vi "CH0_write_byte_data_and_sign_into_mem_no_g_Rev01.vi"(0 "MB data":u8, 1 "UB data":u8, 2 "Sign addrss 8 byte":string, 3 "USB Interface Name":refnum<visa-resource-name>="COM3", 4 "HB data":u8, 5 "LB data":u8, 6 "MB addrss 8 byte":string, 7 "HB addrss 8 byte":string, 8 "Sign data 3 byte":dbl, 9 "WRITE DATA":bool, 10 "Input buffer size":u32=16384, 11 "LB addrss 8 byte":string, 12 "UB addrss 8 byte":string, 13 "error in (no error)":errorcluster, 16 "Enable memory wright":bool) -> (14 "MB data 3 byte":string, 15 "UB data 3 byte":string, 17 "error out":errorcluster, 18 "HB data 3 byte":string, 19 "LB data 3 byte":string)   [LabVIEW 2012]
panel:
  out "Reply":string
  out "T command Bytes sent 5":dbl
  out "T command Bytes sent 4":dbl
  out "T command Bytes sent 3":dbl
  out "T command Bytes sent 2":dbl
  out "T command Bytes sent":dbl
  out "First 'T' Number of bytes written":dbl
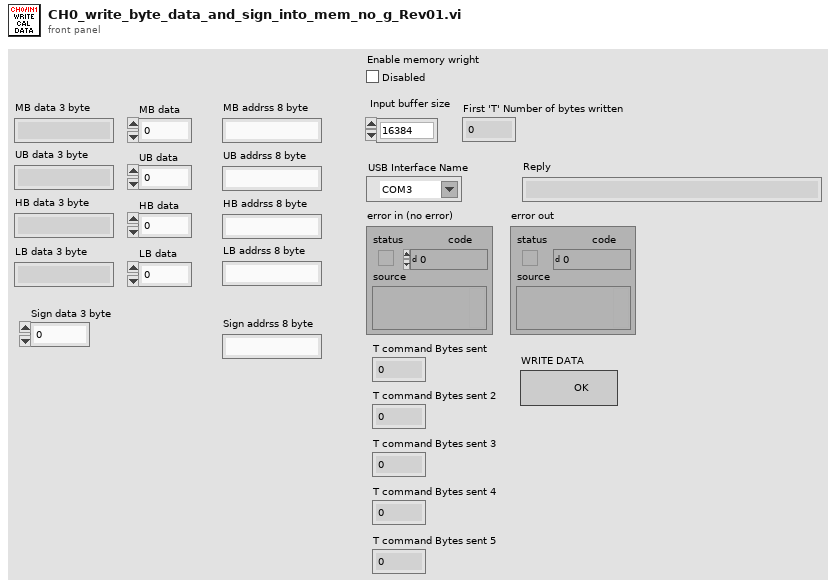
[diagram p1: front panel]
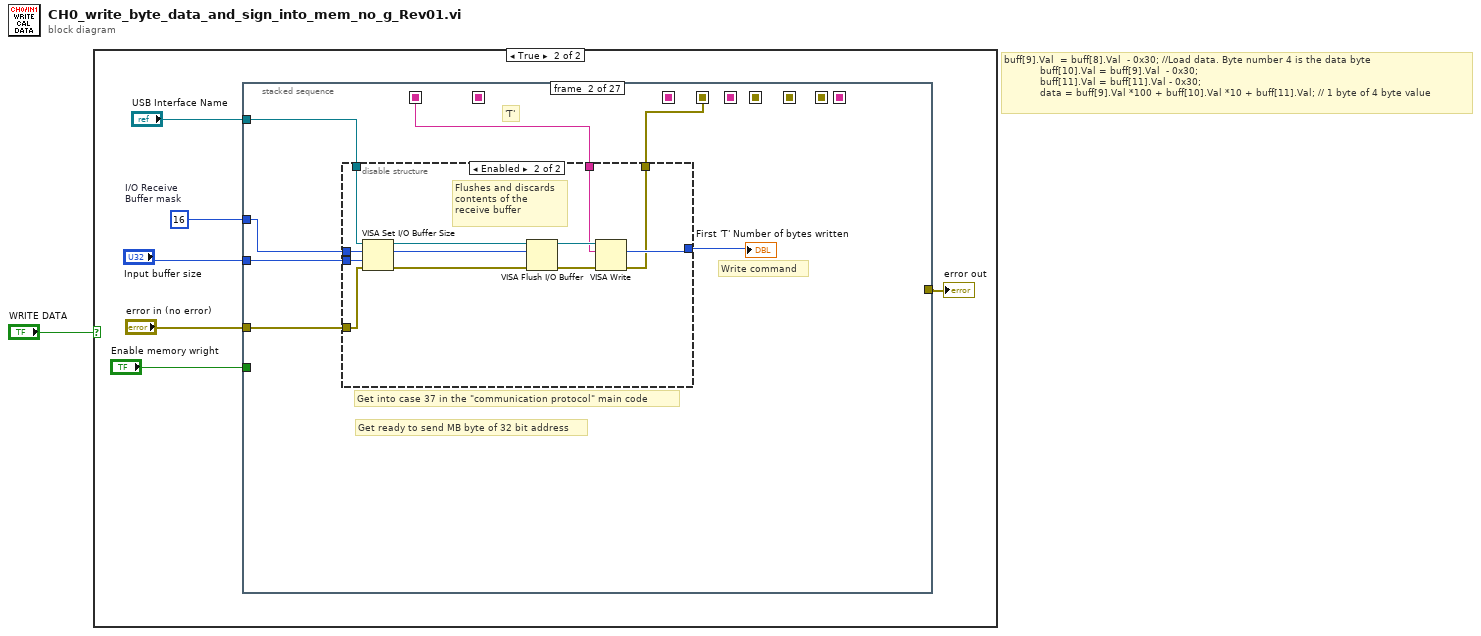
[diagram p0: block diagram]
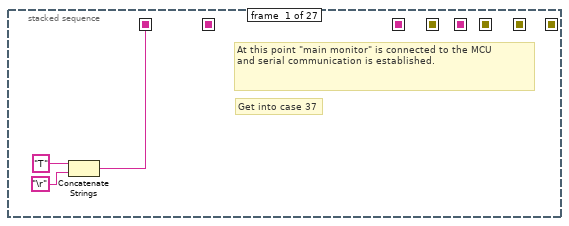
[diagram p3: hidden frame]
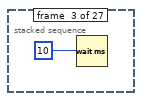
[diagram p5: hidden frame]
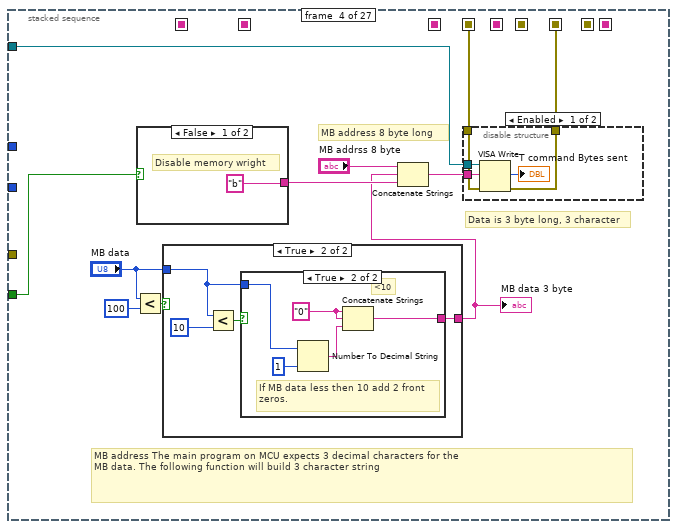
[diagram p6: hidden frame]
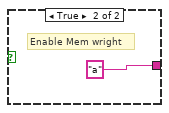
[diagram p7: hidden frame]
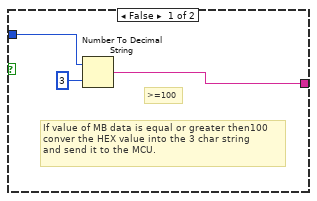
[diagram p8: hidden frame]
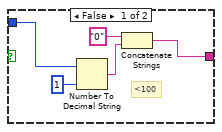
[diagram p9: hidden frame]
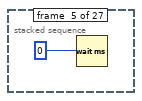
[diagram p11: hidden frame]
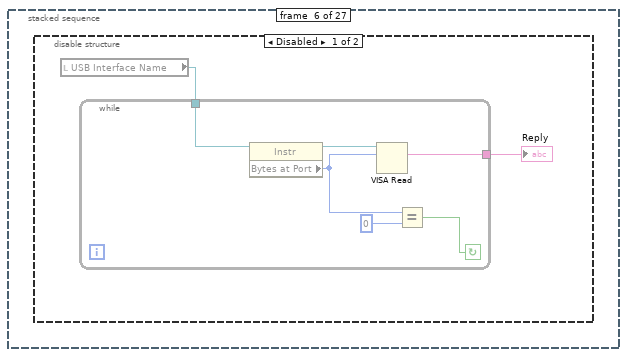
[diagram p12: hidden frame]
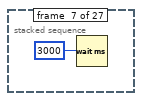
[diagram p14: hidden frame]
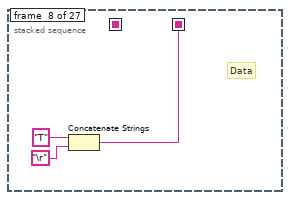
[diagram p15: hidden frame]
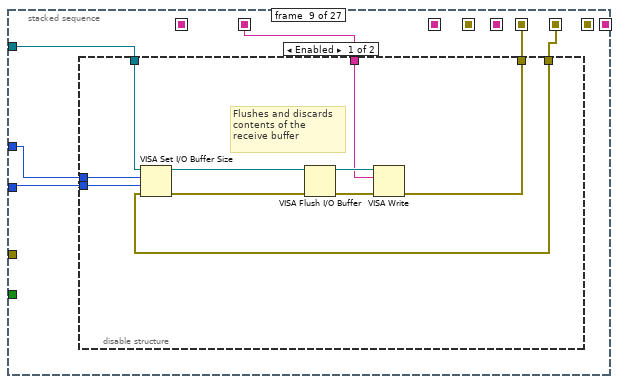
[diagram p16: hidden frame]
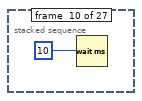
[diagram p18: hidden frame]
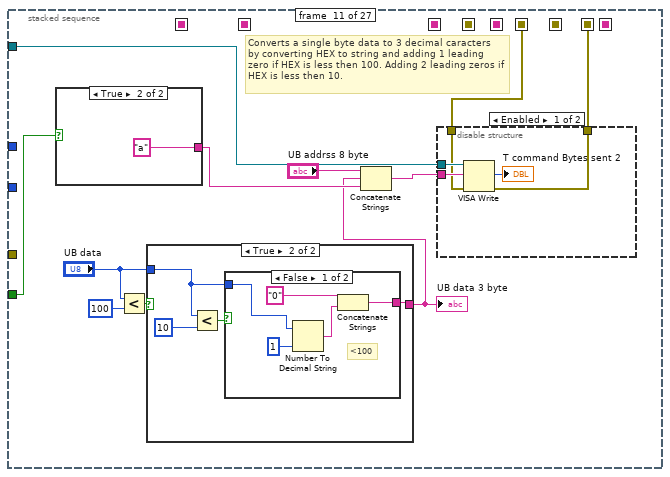
[diagram p19: hidden frame]
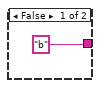
[diagram p20: hidden frame]
diagram:
  # "buff[9].Val  = buff[8].Val  - 0x30; //Load data. Byte number 4 is the data byte           \n            buff[10].Val = buff[9].Val  - 0x30;           \n            buff[11].Val = buff[11].Val - 0x30;               \n            data = buff[9].Val *100 + buff[10].Val *10 + buff[11].Val; // 1 byte of 4 byte value"
  n1 = case shown="True" "WRITE DATA" {
    frame False {
    }
    frame True {
      w5 = u16 16  # I/O Receive Buffer mask
      n2 = stacked-sequence {
        seq-local: [w8 _ _ _ _ _ _ _ _ _ _ _ _ _ _ _ _ _ _ _ _ _ _ _ _ _ _] -> [_ w14 _ _ _ _ _ _ _ _ _ _ _ _ _ _ _ _ _ _ _ _ _ _ _ _ _]
        seq-local: [_ _ _ _ _ _ _ w75 _ _ _ _ _ _ _ _ _ _ _ _ _ _ _ _ _ _ _] -> [_ _ _ _ _ _ _ _ w80 _ _ _ _ _ _ _ _ _ _ _ _ _ _ _ _ _ _]
        seq-local: [_ _ _ _ _ _ _ _ _ _ _ _ w131 _ _ _ _ _ _ _ _ _ _ _ _ _ _] -> [_ _ _ _ _ _ _ _ _ _ _ _ _ w135 _ _ _ _ _ _ _ _ _ _ _ _ _]
        seq-local: [_ _ _ _ _ _ _ _ _ _ _ _ _ _ _ _ _ w182 _ _ _ _ _ _ _ _ _] -> [_ _ _ _ _ _ _ _ _ _ _ _ _ _ _ _ _ _ w185 _ _ _ _ _ _ _ _]
        seq-local: [_ w13 _ _ _ _ _ _ _ _ _ _ _ _ _ _ _ _ _ _ _ _ _ _ _ _ _] -> [_ _ _ w36 _ _ _ _ _ _ _ _ _ _ _ _ _ _ _ _ _ _ _ _ _ _ _]
        seq-local: [_ _ _ w35 _ _ _ _ _ _ _ _ _ _ _ _ _ _ _ _ _ _ _ _ _ _ _] -> [_ _ _ _ _ _ _ _ w79 _ _ _ _ _ _ _ _ _ _ _ _ _ _ _ _ _ _]
        seq-local: [_ _ _ _ _ _ _ _ w78 _ _ _ _ _ _ _ _ _ _ _ _ _ _ _ _ _ _] -> [_ _ _ _ _ _ _ _ _ _ w101 _ _ _ _ _ _ _ _ _ _ _ _ _ _ _ _]
        seq-local: [_ _ _ _ _ _ _ _ _ _ w100 _ _ _ _ _ _ _ _ _ _ _ _ _ _ _ _] -> [_ _ _ _ _ _ _ _ _ _ _ _ _ w134 _ _ _ _ _ _ _ _ _ _ _ _ _]
        seq-local: [_ _ _ _ _ _ _ _ _ _ _ _ _ _ _ _ _ _ _ _ _ _ w235 _ _ _ _] -> [_ _ _ _ _ _ _ _ _ _ _ _ _ _ _ _ _ _ _ _ _ _ _ w238 _ _ _]
        tunnel: "USB Interface Name" -> [_ w17 _ w39 _ _ _ _ w83 _ w102 _ _ w138 _ w155 _ _ w189 _ w207 _ _ w242 _ w262 _]
        tunnel: "error in (no error)" -> [_ w16 _ _ _ _ _ _ _ _ _ _ _ _ _ _ _ _ w187 _ _ _ _ w239 _ _ _]
        tunnel: "Input buffer size" -> [_ w15 _ _ _ _ _ _ w82 _ _ _ _ w136 _ _ _ _ w188 _ _ _ _ w240 _ _ _]
        tunnel: w5 -> [_ w11 _ _ _ _ _ _ w81 _ _ _ _ w137 _ _ _ _ w186 _ _ _ _ w241 _ _ _]
        tunnel: [_ _ _ _ _ _ _ _ _ _ _ _ _ _ _ _ _ _ _ _ w206 _ _ _ _ _ _] -> w4
        tunnel: "Enable memory wright" -> [_ _ _ w33 _ _ _ _ _ _ w97 _ _ _ _ w153 _ _ _ _ w204 _ _ _ _ w254 _]
        frame #0 {
          # "At this point \"main monitor\" is connected to the MCU\nand serial communication is established."
          # "Get into case 37"
          n3 = Concatenate Strings("T", "\r") -> (w8:string)
        }
        frame #1 {
          # "Get ready to send MB byte of 32 bit address"
          # "'T'"
          # "Get into case 37 in the \"communication protocol\" main code"
          # "Write command"
          n4 = disable-structure shown="Enabled" {
            disable-tunnel: w15 -> [_ w24]
            disable-tunnel: w14 -> [_ w23]
            disable-tunnel: w17 -> [_ w22]
            disable-tunnel: w16 -> [_ w21]
            disable-tunnel: [_ w20] -> w12
            disable-tunnel: [_ w19] -> w13
            disable-tunnel: w11 -> [_ w18]
            frame Disabled {
            }
            frame Enabled {
              # "Flushes and discards \ncontents of the \nreceive buffer"
              n5 = VISA Set I/O Buffer Size(VISA resource name=w22, mask (16)=w18, size (4096)=w24, error in (no error)=w21) -> (VISA resource name out=w26:refnum<visa-resource-name>, error out=w25:errorcluster)
              n6 = VISA Flush I/O Buffer(VISA resource name=w26, mask (16)=w18, error in (no error)=w25) -> (VISA resource name out=w28:refnum<visa-resource-name>, error out=w27:errorcluster)
              n7 = VISA Write(VISA resource name=w28, write buffer=w23, error in (no error)=w27) -> (return count=w20:u32, error out=w19:errorcluster)  [unwired: 1 out]
            }
          }
          "First 'T' Number of bytes written" <- w12
        }
        frame #2 {
          n8 = Wait (ms)(milliseconds to wait=10) -> ()  [unwired: 1 out]
        }
        frame #3 {
          # "MB address 8 byte long"
          # "Data is 3 byte long, 3 character"
          # "MB address The main program on MCU expects 3 decimal characters for the \nMB data. The following function will build 3 character string"
          n9 = Less?(x="MB data", y=100) -> (x < y?=w38:bool)
          n10 = case shown="False" w33 {
            tunnel: ["b" "a"] -> w32
            frame False {
              # "Disable memory wright"
            }
            frame True {
              # "Enable Mem wright"
            }
          }
          n11 = case shown="True" w38 {
            tunnel: [w45 w46] -> w30
            tunnel: "MB data" -> [w43 w47]
            frame False {
              # "If value of MB data is equal or greater then100\nconver the HEX value into the 3 char string \nand send it to the MCU."
              # ">=100"
              n12 = Number To Decimal String(number=w43, width (-)=3) -> (decimal integer string=w45:string)
            }
            frame True {
              n13 = Less?(x=w47, y=10) -> (x < y?=w49:bool)
              n14 = case shown="True" w49 {
                tunnel: w47 -> [w52 w55]
                tunnel: [w51 w56] -> w46
                frame False {
                  # "<100"
                  n15 = Number To Decimal String(number=w52, width (-)=1) -> (decimal integer string=w53:string)
                  n16 = Concatenate Strings("0", w53) -> (w51:string)
                }
                frame True {
                  w57 = "0"
                  # "If MB data less then 10 add 2 front\nzeros."
                  # "<10"
                  n17 = Number To Decimal String(number=w55, width (-)=1) -> (decimal integer string=w58:string)
                  n18 = Concatenate Strings(w57, w57, w58) -> (w56:string)
                }
              }
            }
          }
          "MB data 3 byte" <- w30
          n19 = Concatenate Strings("MB addrss 8 byte", w30, w32) -> (w40:string)
          n20 = disable-structure shown="Enabled" {
            disable-tunnel: w40 -> [w63 _]
            disable-tunnel: w39 -> [w62 _]
            disable-tunnel: w36 -> [w61 _]
            disable-tunnel: [w60 _] -> w35
            frame Enabled {
              n21 = VISA Write(VISA resource name=w62, write buffer=w63, error in (no error)=w61) -> (return count=→"T command Bytes sent":u32, error out=w60:errorcluster)  [unwired: 1 out]
            }
            frame Disabled {
            }
          }
        }
        frame #4 {
          n22 = Wait (ms)(milliseconds to wait=0) -> ()  [unwired: 1 out]
        }
        frame #5 {
          n23 = disable-structure shown="Disabled" {
            frame Disabled {
              n24 = local read "USB Interface Name"() -> (w67:refnum<visa-resource-name>)
              n25 = while {
                tunnel: w67 -> [w69]
                tunnel: [w68] -> w66
                stop <- w70 continue-if-true
                n26 = property class="Instr"(reference=w69) -> (reference out=w73:refnum<visa-resource-name>, "Bytes at Port"=w72:u32)  [unwired: 1 in, 1 out]
                n27 = VISA Read(VISA resource name=w73, byte count=w72) -> (read buffer=w68:string)  [unwired: 1 in, 3 out]
                n28 = Equal?(x=w72, y=0) -> (x = y?=w70:bool)
              }
              "Reply" <- w66
            }
            frame Enabled {
            }
          }
        }
        frame #6 {
          n29 = Wait (ms)(milliseconds to wait=3000) -> ()  [unwired: 1 out]
        }
        frame #7 {
          # "Data"
          n30 = Concatenate Strings("T", "\r") -> (w75:string)
        }
        frame #8 {
          n31 = disable-structure shown="Enabled" {
            disable-tunnel: w83 -> [w89 _]
            disable-tunnel: w82 -> [w88 _]
            disable-tunnel: w81 -> [w87 _]
            disable-tunnel: w80 -> [w86 _]
            disable-tunnel: w79 -> [w85 _]
            disable-tunnel: [w84 _] -> w78
            frame Enabled {
              # "Flushes and discards \ncontents of the \nreceive buffer"
              n32 = VISA Set I/O Buffer Size(VISA resource name=w89, mask (16)=w87, size (4096)=w88, error in (no error)=w85) -> (VISA resource name out=w91:refnum<visa-resource-name>, error out=w90:errorcluster)
              n33 = VISA Flush I/O Buffer(VISA resource name=w91, error in (no error)=w90) -> (VISA resource name out=w93:refnum<visa-resource-name>, error out=w92:errorcluster)  [unwired: 1 in]
              n34 = VISA Write(VISA resource name=w93, write buffer=w86, error in (no error)=w92) -> (error out=w84:errorcluster)  [unwired: 2 out]
            }
            frame Disabled {
            }
          }
        }
        frame #9 {
          n35 = Wait (ms)(milliseconds to wait=10) -> ()  [unwired: 1 out]
        }
        frame #10 {
          # "Converts a single byte data to 3 decimal caracters\nby converting HEX to string and adding 1 leading zero if HEX is less then 100. Adding 2 leading zeros if HEX is less then 10."
          n36 = case shown="True" w97 {
            tunnel: ["b" "a"] -> w98
            frame False {
            }
            frame True {
            }
          }
          n37 = Less?(x="UB data", y=100) -> (x < y?=w104:bool)
          n38 = case shown="True" w104 {
            tunnel: [w110 w111] -> w95
            tunnel: "UB data" -> [w108 w112]
            frame False {
              # ">=100"
              n39 = Number To Decimal String(number=w108, width (-)=3) -> (decimal integer string=w110:string)
            }
            frame True {
              n40 = Less?(x=w112, y=10) -> (x < y?=w114:bool)
              n41 = case shown="False" w114 {
                tunnel: w112 -> [w116 w120]
                tunnel: [w115 w121] -> w111
                frame False {
                  # "<100"
                  n42 = Number To Decimal String(number=w116, width (-)=1) -> (decimal integer string=w117:string)
                  n43 = Concatenate Strings("0", w117) -> (w115:string)
                }
                frame True {
                  w122 = "0"
                  # "<10"
                  n44 = Number To Decimal String(number=w120, width (-)=1) -> (decimal integer string=w123:string)
                  n45 = Concatenate Strings(w122, w122, w123) -> (w121:string)
                }
              }
            }
          }
          "UB data 3 byte" <- w95
          n46 = Concatenate Strings("UB addrss 8 byte", w95, w98) -> (w105:string)
          n47 = disable-structure shown="Enabled" {
            disable-tunnel: w105 -> [w128 _]
            disable-tunnel: w102 -> [w127 _]
            disable-tunnel: w101 -> [w126 _]
            disable-tunnel: [w125 _] -> w100
            frame Enabled {
              n48 = VISA Write(VISA resource name=w127, write buffer=w128, error in (no error)=w126) -> (return count=→"T command Bytes sent 2":u32, error out=w125:errorcluster)  [unwired: 1 out]
            }
            frame Disabled {
            }
          }
        }
        frame #11 {
          n49 = Wait (ms)(milliseconds to wait=3000) -> ()  [unwired: 1 out]
        }
        frame #12 {
          n50 = Concatenate Strings("T", "\r") -> (w131:string)
        }
        frame #13 {
          n51 = disable-structure shown="Enabled" {
            disable-tunnel: w138 -> [w143 _]
            disable-tunnel: w137 -> [w142 _]
            disable-tunnel: w136 -> [w141 _]
            disable-tunnel: w135 -> [w140 _]
            disable-tunnel: w134 -> [w139 _]
            frame Enabled {
              # "Flushes and discards \ncontents of the \nreceive buffer"
              n52 = VISA Set I/O Buffer Size(VISA resource name=w143, mask (16)=w142, size (4096)=w141, error in (no error)=w139) -> (VISA resource name out=w145:refnum<visa-resource-name>, error out=w144:errorcluster)
              n53 = VISA Flush I/O Buffer(VISA resource name=w145, error in (no error)=w144) -> (VISA resource name out=w147:refnum<visa-resource-name>, error out=w146:errorcluster)  [unwired: 1 in]
              n54 = VISA Write(VISA resource name=w147, write buffer=w140, error in (no error)=w146) -> ()  [unwired: 3 out]
            }
            frame Disabled {
            }
          }
        }
        frame #14 {
          n55 = Wait (ms)(milliseconds to wait=10) -> ()  [unwired: 1 out]
        }
        frame #15 {
          # "Converts a single byte data to 3 decimal caracters\nby converting HEX to string and adding 1 leading zero if HEX is less then 100. Adding 2 leading zeros if HEX is less then 10."
          n56 = case shown="True" w153 {
            tunnel: ["b" "a"] -> w152
            frame False {
            }
            frame True {
            }
          }
          n57 = Less?(x="HB data", y=100) -> (x < y?=w157:bool)
          n58 = case shown="True" w157 {
            tunnel: [w163 w164] -> w149
            tunnel: "HB data" -> [w161 w165]
            frame False {
              # ">=100"
              n59 = Number To Decimal String(number=w161, width (-)=3) -> (decimal integer string=w163:string)
            }
            frame True {
              n60 = Less?(x=w165, y=10) -> (x < y?=w167:bool)
              n61 = case shown="False" w167 {
                tunnel: w165 -> [w169 w173]
                tunnel: [w168 w174] -> w164
                frame False {
                  # "<100"
                  n62 = Number To Decimal String(number=w169, width (-)=1) -> (decimal integer string=w170:string)
                  n63 = Concatenate Strings("0", w170) -> (w168:string)
                }
                frame True {
                  w175 = "0"
                  # "<10"
                  n64 = Number To Decimal String(number=w173, width (-)=1) -> (decimal integer string=w176:string)
                  n65 = Concatenate Strings(w175, w175, w176) -> (w174:string)
                }
              }
            }
          }
          "HB data 3 byte" <- w149
          n66 = Number To Decimal String(number="HB data", width (-)=3) -> ()  [unwired: 1 out]
          n67 = Concatenate Strings("HB addrss 8 byte", w149, w152) -> (w158:string)
          n68 = disable-structure shown="Enabled" {
            disable-tunnel: w158 -> [w179 _]
            disable-tunnel: w155 -> [w178 _]
            frame Enabled {
              n69 = VISA Write(VISA resource name=w178, write buffer=w179) -> (return count=→"T command Bytes sent 3":u32)  [unwired: 1 in, 2 out]
            }
            frame Disabled {
            }
          }
        }
        frame #16 {
          n70 = Wait (ms)(milliseconds to wait=5000) -> ()  [unwired: 1 out]
        }
        frame #17 {
          # "Get into case 37"
          n71 = Concatenate Strings("T", "\r") -> (w182:string)
        }
        frame #18 {
          # "Get into case 37 in the communication protocol"
          # "Write command"
          n72 = disable-structure shown="Enabled" {
            disable-tunnel: w188 -> [w195 _]
            disable-tunnel: w185 -> [w194 _]
            disable-tunnel: w189 -> [w193 _]
            disable-tunnel: w187 -> [w192 _]
            disable-tunnel: [w191 _] -> _
            disable-tunnel: w186 -> [w190 _]
            frame Enabled {
              # "Flushes and discards \ncontents of the \nreceive buffer"
              n73 = VISA Set I/O Buffer Size(VISA resource name=w193, mask (16)=w190, size (4096)=w195, error in (no error)=w192) -> (VISA resource name out=w197:refnum<visa-resource-name>, error out=w196:errorcluster)
              n74 = VISA Flush I/O Buffer(VISA resource name=w197, error in (no error)=w196) -> (VISA resource name out=w199:refnum<visa-resource-name>, error out=w198:errorcluster)  [unwired: 1 in]
              n75 = VISA Write(VISA resource name=w199, write buffer=w194, error in (no error)=w198) -> (return count=w191:u32)  [unwired: 2 out]
            }
            frame Disabled {
            }
          }
        }
        frame #19 {
          n76 = Wait (ms)(milliseconds to wait=10) -> ()  [unwired: 1 out]
        }
        frame #20 {
          # "The main program on MCU expects 3 decimal characters for the \nMB data. The following function will build 3 character string"
          n77 = case shown="True" w204 {
            tunnel: ["b" "a"] -> w203
            frame False {
            }
            frame True {
              # "Enable memory wright"
            }
          }
          n78 = Number To Decimal String(number="LB data") -> ()  [unwired: 1 in, 1 out]
          n79 = Less?(x="LB data", y=100) -> (x < y?=w209:bool)
          n80 = case shown="True" w209 {
            tunnel: [w215 w216] -> w202
            tunnel: "LB data" -> [w213 w217]
            frame False {
              # ">=100"
              n81 = Number To Decimal String(number=w213, width (-)=3) -> (decimal integer string=w215:string)
            }
            frame True {
              n82 = Less?(x=w217, y=10) -> (x < y?=w219:bool)
              n83 = case shown="True" w219 {
                tunnel: w217 -> [w221 w225]
                tunnel: [w220 w226] -> w216
                frame False {
                  # "<100"
                  n84 = Number To Decimal String(number=w221, width (-)=1) -> (decimal integer string=w222:string)
                  n85 = Concatenate Strings("0", w222) -> (w220:string)
                }
                frame True {
                  w227 = "0"
                  # "<10"
                  n86 = Number To Decimal String(number=w225, width (-)=1) -> (decimal integer string=w228:string)
                  n87 = Concatenate Strings(w227, w227, w228) -> (w226:string)
                }
              }
            }
          }
          "LB data 3 byte" <- w202
          n88 = Concatenate Strings("LB addrss 8 byte", w202, w203) -> (w210:string)
          n89 = disable-structure shown="Enabled" {
            disable-tunnel: w210 -> [w232 _]
            disable-tunnel: w207 -> [w231 _]
            disable-tunnel: [w230 _] -> w206
            frame Enabled {
              n90 = VISA Write(VISA resource name=w231, write buffer=w232) -> (return count=→"T command Bytes sent 4":u32, error out=w230:errorcluster)  [unwired: 1 in, 1 out]
            }
            frame Disabled {
            }
          }
        }
        frame #21 {
          n91 = Wait (ms)(milliseconds to wait=5000) -> ()  [unwired: 1 out]
        }
        frame #22 {
          # "Send sign"
          n92 = Concatenate Strings("T", "\r") -> (w235:string)
        }
        frame #23 {
          # "Get into case 37 in the communication protocol"
          # "Write command"
          n93 = disable-structure shown="Enabled" {
            disable-tunnel: w240 -> [w248 _]
            disable-tunnel: w238 -> [w247 _]
            disable-tunnel: w242 -> [w246 _]
            disable-tunnel: w239 -> [w245 _]
            disable-tunnel: [w244 _] -> _
            disable-tunnel: w241 -> [w243 _]
            frame Enabled {
              # "Flushes and discards \ncontents of the \nreceive buffer"
              n94 = VISA Set I/O Buffer Size(VISA resource name=w246, mask (16)=w243, size (4096)=w248, error in (no error)=w245) -> (VISA resource name out=w250:refnum<visa-resource-name>, error out=w249:errorcluster)
              n95 = VISA Flush I/O Buffer(VISA resource name=w250, error in (no error)=w249) -> (VISA resource name out=w252:refnum<visa-resource-name>, error out=w251:errorcluster)  [unwired: 1 in]
              n96 = VISA Write(VISA resource name=w252, write buffer=w247, error in (no error)=w251) -> (return count=w244:u32)  [unwired: 2 out]
            }
            frame Disabled {
            }
          }
        }
        frame #24 {
          n97 = Wait (ms)(milliseconds to wait=10) -> ()  [unwired: 1 out]
        }
        frame #25 {
          w259 = "0"
          # "001 or 000"
          # "<10"
          n98 = case shown="True" w254 {
            tunnel: ["b" "a"] -> w255
            frame False {
            }
            frame True {
            }
          }
          n99 = Number To Decimal String(number="Sign data 3 byte", width (-)=1) -> (decimal integer string=w260:string)
          n100 = Concatenate Strings(w259, w259, w260) -> (w257:string)
          n101 = Concatenate Strings("Sign addrss 8 byte", w257, w255) -> (w263:string)
          n102 = disable-structure shown="Enabled" {
            disable-tunnel: w263 -> [w268 _]
            disable-tunnel: w262 -> [w267 _]
            disable-tunnel: [w266 _] -> _
            frame Enabled {
              n103 = VISA Write(VISA resource name=w267, write buffer=w268) -> (return count=→"T command Bytes sent 5":u32, error out=w266:errorcluster)  [unwired: 1 in, 1 out]
            }
            frame Disabled {
            }
          }
        }
        frame #26 {
          n104 = Wait (ms)(milliseconds to wait=5000) -> ()  [unwired: 1 out]
        }
      }
      "error out" <- w4
    }
  }
